vi "Untitled 1.vi"() -> ()   [LabVIEW 2019]
panel:
  in  "stop":bool
  in  "milliseconds to wait":u32=100
  out "Arbitrary Signal":waveform(dbl)(graph)
  out "x+y":dbl
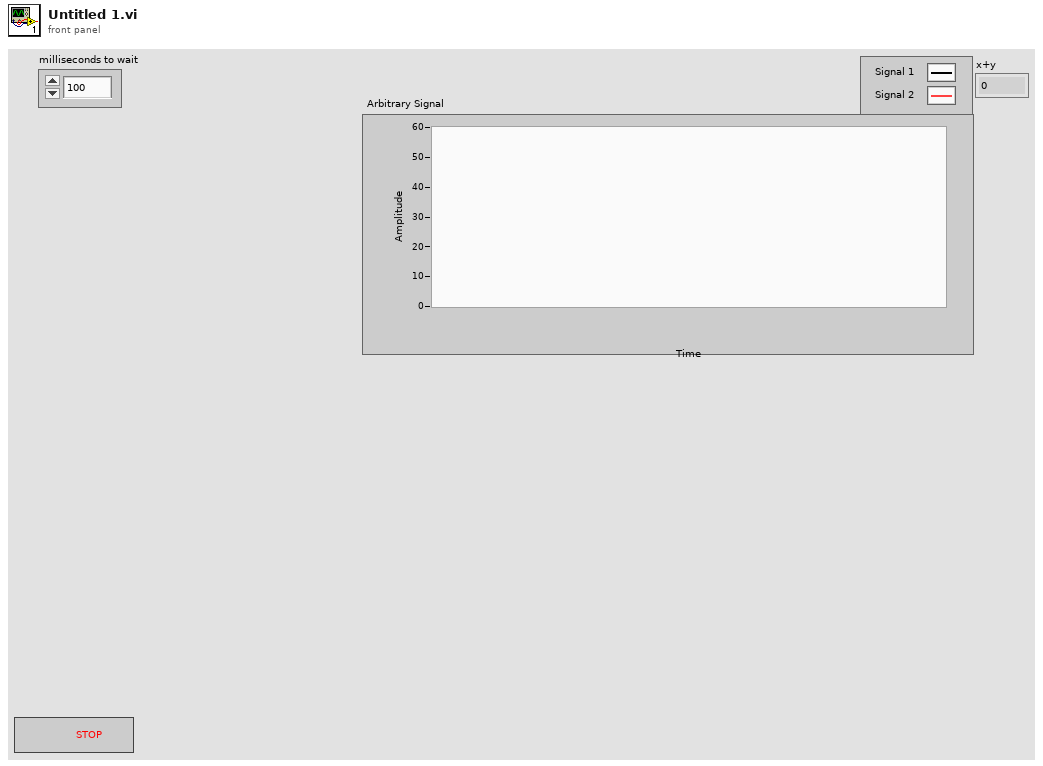
[diagram p1: front panel]
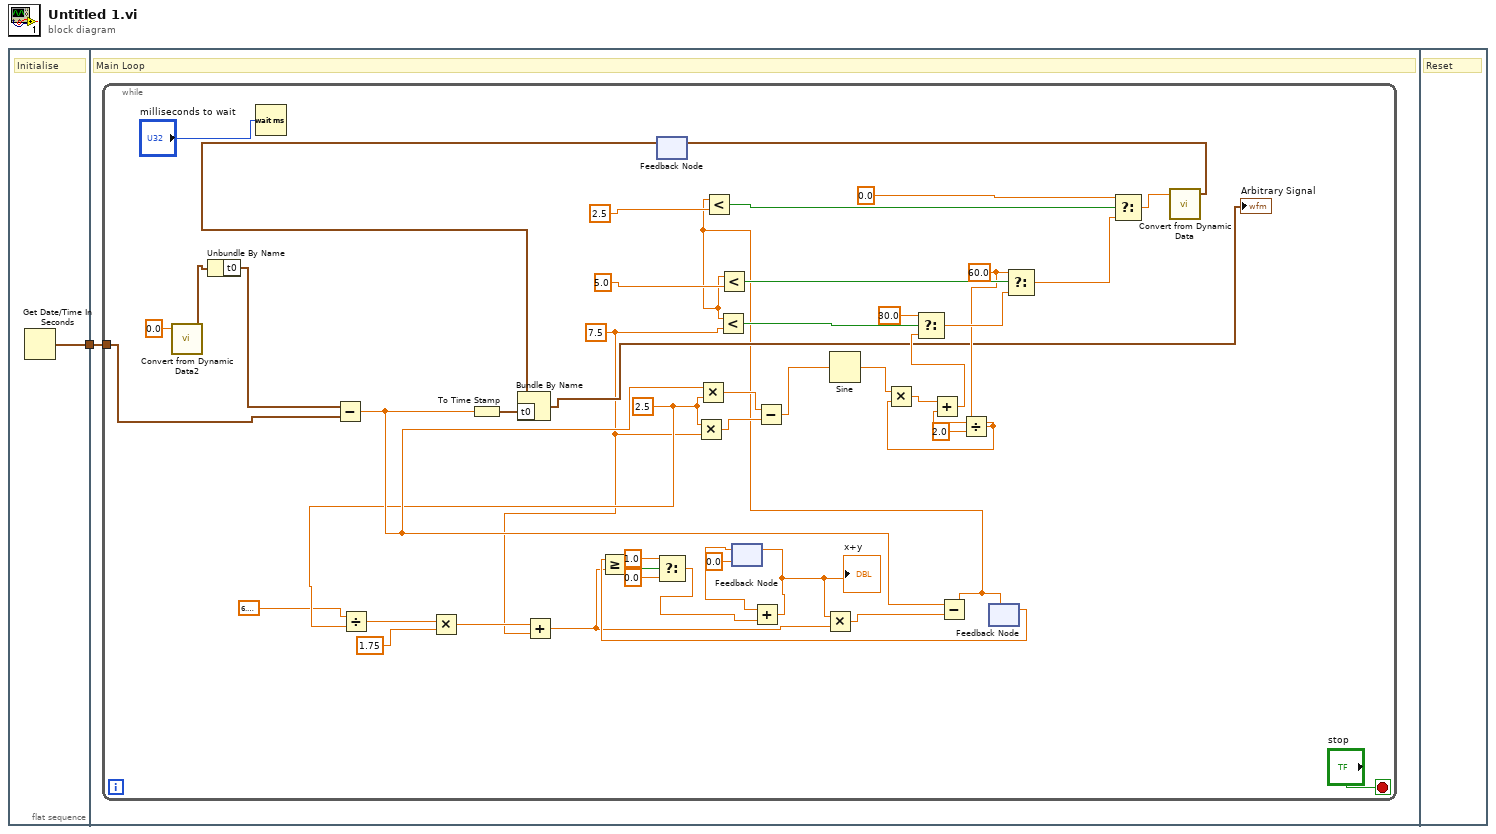
[diagram p0: block diagram]
diagram:
  n1 = flat-sequence {
    tunnel: [w2] -> w1
    tunnel: w1 -> [w3]
    frame #0 {
      # "Initialise"
      n2 = Get Date/Time In Seconds() -> (seconds since 1Jan1904=w2:timestamp)
    }
    frame #1 {
      # "Main Loop"
      n3 = while {
        tunnel: w3 -> [w44]
        stop <- "stop" stop-if-true
        w16 = 2.5 ("y")
        w36 = 60.0 ("t")
        w5 = 7.5 ("number")
        n4 = call "Convert from Dynamic Data2"("Dynamic Data Type"=0.0) -> ("Waveform"=w9:waveform(dbl))  [unwired: 3 in]
        n5 = Unbundle By Name ("Get Waveform Components")(w9) -> ("t0"=w12:timestamp)
        n6 = Wait (ms)(milliseconds to wait="milliseconds to wait") -> ()  [unwired: 1 out]
        n7 = Subtract(x=w12, y=w44) -> (x-y=w21:dbl)
        n8 = Divide(x=6.283185307179586, y=w16) -> (x/y=w15:dbl)
        n9 = Multiply(x=w15, y=1.75) -> (x*y=w17:dbl)
        n10 = To Time Stamp(1:w21) -> (0:w48:timestamp)
        n11 = Add(x=w17, y=w5) -> (x+y=w19:dbl)
        n12 = feedback #1() -> (w10:waveform(dbl))  [unwired: 1 in]
        n13 = Bundle By Name ("Build Waveform")(cluster=w10, "t0"=w48) -> (→"Arbitrary Signal":waveform(dbl))
        n14 = Multiply(x=w16, y=w5) -> (x*y=w32:dbl)
        n15 = Multiply(x=w21, y=w16) -> (x*y=w31:dbl)
        n16 = feedback #2(0.0) -> (w22:dbl)
        n17 = Subtract(x=w31, y=w32) -> (x-y=w33:dbl)
        n18 = Sine(x=w33) -> (sin(x)=w39:dbl)
        n19 = Divide(x=w36, y=2.0) -> (x/y=w34:dbl)
        n20 = Multiply(x=w39, y=w34) -> (x*y=w38:dbl)
        n21 = Add(x=w38, y=w34) -> (x+y=w37:dbl)
        n22 = feedback #3() -> (w20:dbl)  [unwired: 1 in]
        n23 = Greater Or Equal?(x=w20, y=w19) -> (x >= y?=w29:bool)
        n24 = Select(t=1.0, s=w29, f=0.0) -> (s? t:f=w23:dbl)
        n25 = Add(x=w22, y=w23) -> (x+y=w24:dbl)
        "x+y" <- w24
        n26 = feedback-in #2(w24) -> ()
        n27 = Multiply(x=w24, y=w19) -> (x*y=w27:dbl)
        n28 = Subtract(x=w21, y=w27) -> (x-y=w4:dbl)
        n29 = Less?(x=w4, y=2.5 ("number")) -> (x < y?=w47:bool)
        n30 = Less?(x=w4, y=w5) -> (x < y?=w45:bool)
        n31 = Less?(x=w4, y=5.0 ("number")) -> (x < y?=w46:bool)
        n32 = Select(t=30.0, s=w45, f=w37) -> (s? t:f=w41:dbl)
        n33 = feedback-in #3(w4) -> ()
        n34 = Select(t=w36, s=w46, f=w41) -> (s? t:f=w42:dbl)
        n35 = Select(t=0.0, s=w47, f=w42) -> (s? t:f=w30:dbl)
        n36 = call "Convert from Dynamic Data"("Dynamic Data Type"=w30) -> ("Waveform"=w11:waveform(dbl))  [unwired: 3 in]
        n37 = feedback-in #1(w11) -> ()
      }
    }
    frame #2 {
      # "Reset"
    }
  }
